vi "ReadIOValues gas.vi"(3 "error in":errorcluster, 5 "Output - Cluster gas":T1 {"GM TS-2[°C]" format="%.2g"; "GM TS-1 [°C]" format="%.4g"; "GM DS-1 [bar]" format="%.4g"; "GM DS-2 [bar]" format="%.2g"; "GM GZ-1 [imp]" format="%.2g"}) -> (0 "error out":errorcluster, 2 "Output - Cluster gas":T1 {"GM TS-2[°C]" format="%.2g"; "GM TS-1 [°C]" format="%.4g"; "GM DS-1 [bar]" format="%.4g"; "GM DS-2 [bar]" format="%.2g"; "GM GZ-1 [imp]" format="%.2g"})   [LabVIEW 2011]
uses:
  Output - Cluster gas.ctl
  gas_values.ctl
  <vilib>/functionblocks/Counter/Count Up/Count Up.vi
  <vilib>/functionblocks/FB Core/FB Core.xnode
  <vilib>/functionblocks/NI_FunctionBlock Libraries.lvlib
panel:
  # "qualitätsmessung"
  # "quantitätsmessung"
  # "qualitätsmessung"
  # "quantitätsmessung"
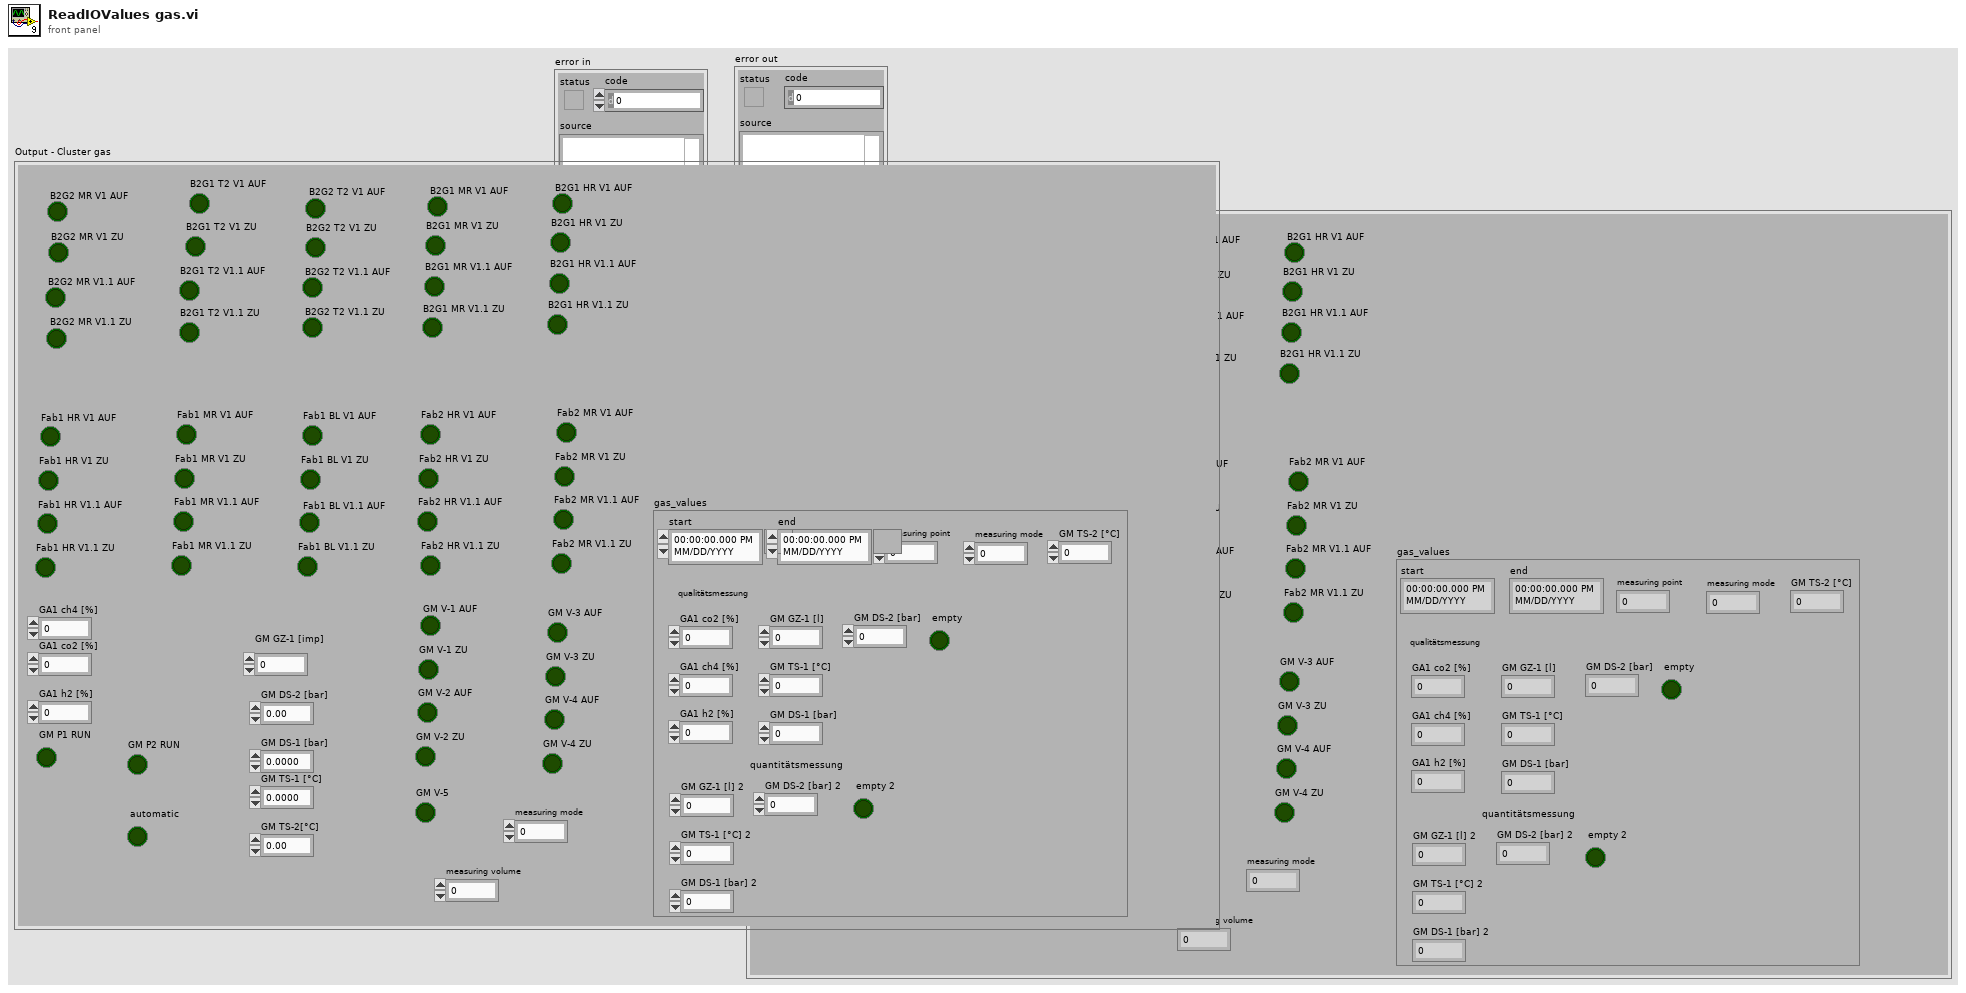
[diagram p1: front panel]
types:
  T1 = typedef "Output - Cluster gas.ctl" = cluster{"B2G2 MR V1.1 AUF":bool, "B2G2 MR V1.1 ZU":bool, "B2G2 MR V1 AUF":bool, "B2G2 MR V1 ZU":bool, "B2G1 T2 V1 AUF":bool, "B2G1 T2 V1 ZU":bool, "B2G1 T2 V1.1 AUF":bool, "B2G1 T2 V1.1 ZU":bool, "B2G2 T2 V1 AUF":bool, "B2G2 T2 V1 ZU":bool, "B2G2 T2 V1.1 ZU":bool, "B2G2 T2 V1.1 AUF":bool, "B2G1 MR V1 AUF":bool, "B2G1 MR V1 ZU":bool, "B2G1 MR V1.1 AUF":bool, "B2G1 MR V1.1 ZU":bool, "B2G1 HR V1 AUF":bool, "B2G1 HR V1 ZU":bool, "B2G1 HR V1.1 AUF":bool, "B2G1 HR V1.1 ZU":bool, "Fab1 HR V1 AUF":bool, "Fab1 HR V1 ZU":bool, "Fab1 HR V1.1 AUF":bool, "Fab1 HR V1.1 ZU":bool, "Fab1 MR V1 AUF":bool, "Fab1 MR V1 ZU":bool, "Fab1 MR V1.1 AUF":bool, "Fab1 MR V1.1 ZU":bool, "Fab1 BL V1 AUF":bool, "Fab1 BL V1 ZU":bool, "Fab1 BL V1.1 AUF":bool, "Fab1 BL V1.1 ZU":bool, "Fab2 HR V1 AUF":bool, "Fab2 HR V1 ZU":bool, "Fab2 HR V1.1 AUF":bool, "Fab2 HR V1.1 ZU":bool, "Fab2 MR V1 AUF":bool, "Fab2 MR V1 ZU":bool, "Fab2 MR V1.1 AUF":bool, "Fab2 MR V1.1 ZU":bool, "GA1 ch4 [%]":dbl, "GA1 co2 [%]":dbl, "GA1 h2 [%]":dbl, "GM P1 RUN":bool, "GM V-1 AUF":bool, "GM V-1 ZU":bool, "GM V-2 AUF":bool, "GM V-2 ZU":bool, "GM V-3 AUF":bool, "GM V-3 ZU":bool, "GM V-4 AUF":bool, "GM V-4 ZU":bool, "GM P2 RUN":bool, "GM GZ-1 [imp]":u32, "GM DS-2 [bar]":dbl, "GM DS-1 [bar]":dbl, "GM TS-1 [°C]":dbl, "GM TS-2[°C]":dbl, "gas_values":T2, "measuring mode":u8, "GM V-5":bool, "measuring volume":dbl, "automatic":bool}
  T2 = typedef "gas_values.ctl" = cluster{"start":timestamp, "GM DS-2 [bar]":dbl, "GA1 ch4 [%]":dbl, "GA1 co2 [%]":dbl, "GA1 h2 [%]":dbl, "GM DS-1 [bar]":dbl, "GM TS-1 [°C]":dbl, "GM TS-2 [°C]":dbl, "GM GZ-1 [l]":dbl, "measuring point":u8, "end":timestamp, "empty":bool, "GM GZ-1 [l] 2":dbl, "GM TS-1 [°C] 2":dbl, "GM DS-1 [bar] 2":dbl, "GM DS-2 [bar] 2":dbl, "empty 2":bool, "measuring mode":u8}
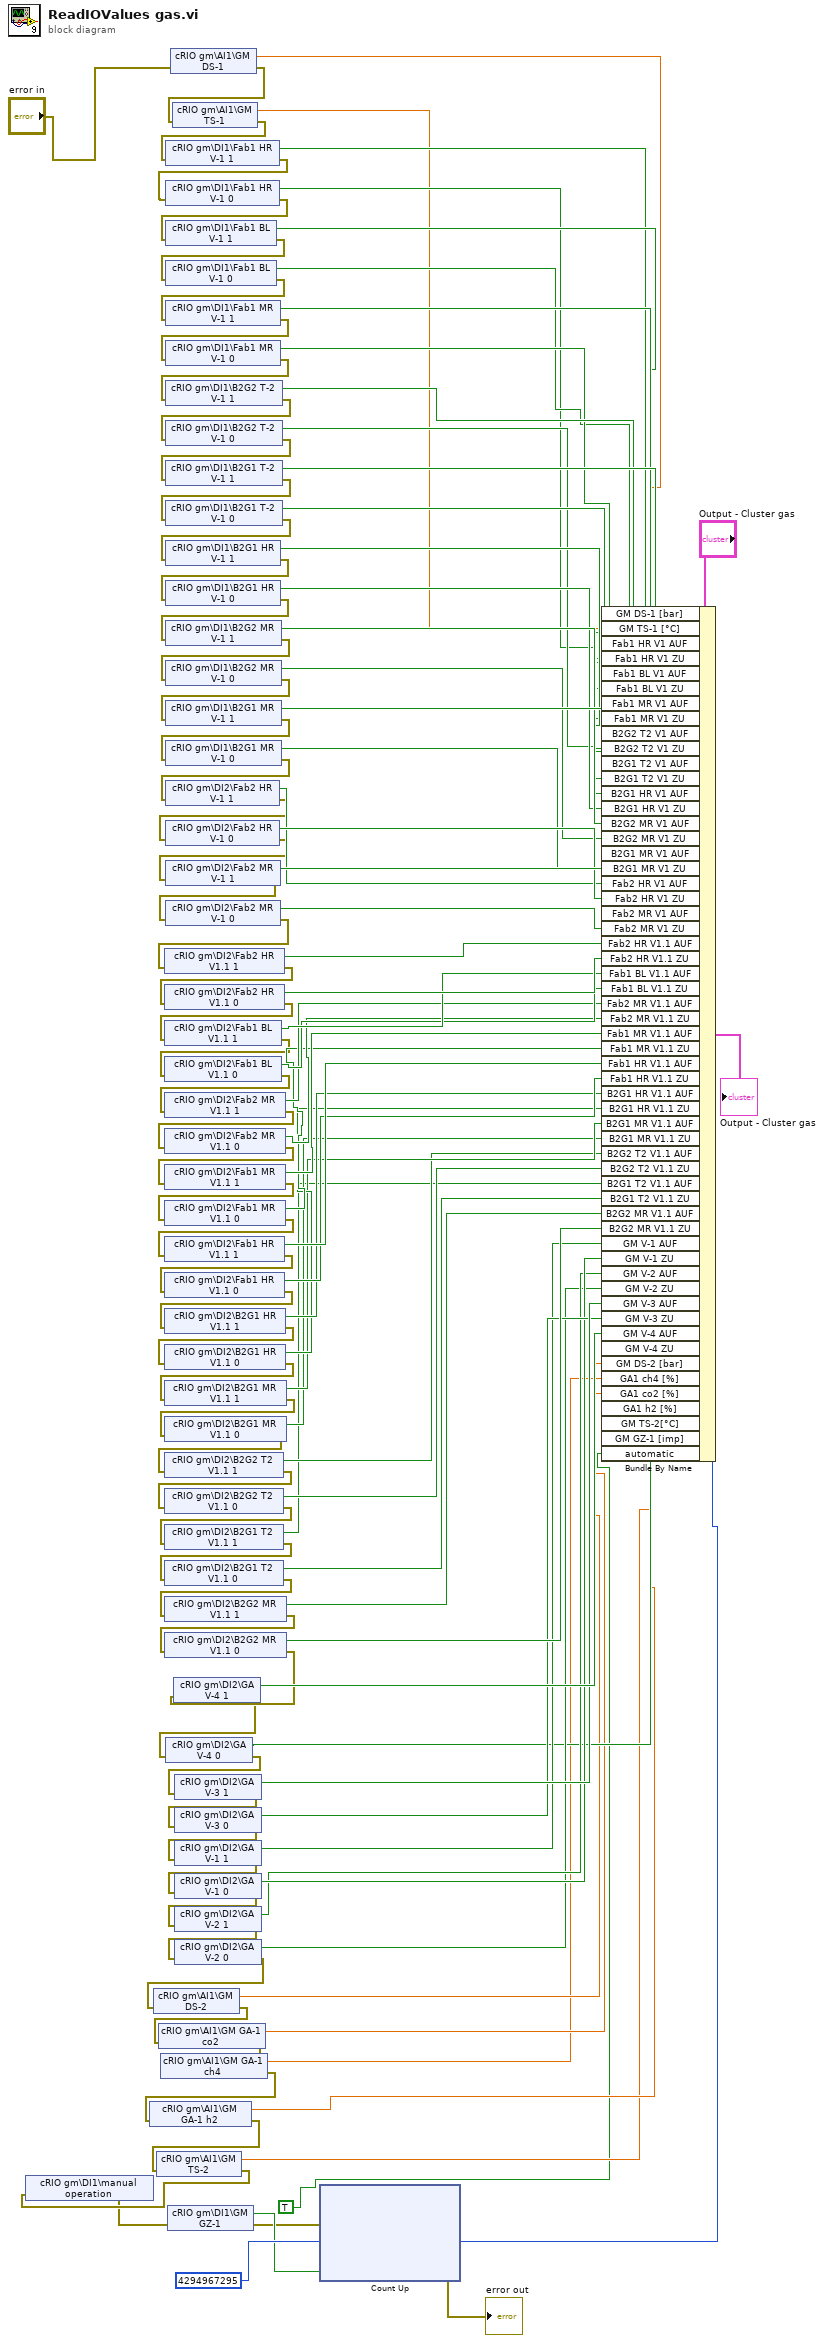
[diagram p0: block diagram]
diagram:
  n1 = shared-variable "cRIO gm\\AI1\\GM DS-1"(error in="error in") -> (w5:dbl, error out=w7:errorcluster)
  n2 = shared-variable "cRIO gm\\AI1\\GM TS-1"(error in=w7) -> (w4:dbl, error out=w6:errorcluster)
  n3 = shared-variable "cRIO gm\\DI1\\Fab1 HR V-1 1"(error in=w6) -> (w9:bool, error out=w44:errorcluster)
  n4 = shared-variable "cRIO gm\\DI1\\Fab1 HR V-1 0"(error in=w44) -> (w10:bool, error out=w43:errorcluster)
  n5 = shared-variable "cRIO gm\\DI1\\Fab1 BL V-1 1"(error in=w43) -> (w11:bool, error out=w42:errorcluster)
  n6 = shared-variable "cRIO gm\\DI1\\Fab1 BL V-1 0"(error in=w42) -> (w12:bool, error out=w41:errorcluster)
  n7 = shared-variable "cRIO gm\\DI1\\Fab1 MR V-1 1"(error in=w41) -> (w13:bool, error out=w40:errorcluster)
  n8 = shared-variable "cRIO gm\\DI1\\Fab1 MR V-1 0"(error in=w40) -> (w14:bool, error out=w39:errorcluster)
  n9 = shared-variable "cRIO gm\\DI1\\B2G2 T-2 V-1 1"(error in=w39) -> (w15:bool, error out=w38:errorcluster)
  n10 = shared-variable "cRIO gm\\DI1\\B2G2 T-2 V-1 0"(error in=w38) -> (w16:bool, error out=w37:errorcluster)
  n11 = shared-variable "cRIO gm\\DI1\\B2G1 T-2 V-1 1"(error in=w37) -> (w17:bool, error out=w36:errorcluster)
  n12 = shared-variable "cRIO gm\\DI1\\B2G1 T-2 V-1 0"(error in=w36) -> (w18:bool, error out=w35:errorcluster)
  n13 = shared-variable "cRIO gm\\DI1\\B2G1 HR V-1 1"(error in=w35) -> (w19:bool, error out=w34:errorcluster)
  n14 = shared-variable "cRIO gm\\DI1\\B2G1 HR V-1 0"(error in=w34) -> (w20:bool, error out=w33:errorcluster)
  n15 = shared-variable "cRIO gm\\DI1\\B2G2 MR V-1 1"(error in=w33) -> (w21:bool, error out=w32:errorcluster)
  n16 = shared-variable "cRIO gm\\DI1\\B2G2 MR V-1 0"(error in=w32) -> (w22:bool, error out=w31:errorcluster)
  n17 = shared-variable "cRIO gm\\DI1\\B2G1 MR V-1 1"(error in=w31) -> (w24:bool, error out=w30:errorcluster)
  n18 = shared-variable "cRIO gm\\DI1\\B2G1 MR V-1 0"(error in=w30) -> (w23:bool, error out=w29:errorcluster)
  n19 = shared-variable "cRIO gm\\DI2\\Fab2 HR V-1 1"(error in=w29) -> (w45:bool, error out=w28:errorcluster)
  n20 = shared-variable "cRIO gm\\DI2\\Fab2 HR V-1 0"(error in=w28) -> (w46:bool, error out=w27:errorcluster)
  n21 = shared-variable "cRIO gm\\DI2\\Fab2 MR V-1 1"(error in=w27) -> (w47:bool, error out=w26:errorcluster)
  n22 = shared-variable "cRIO gm\\DI2\\Fab2 MR V-1 0"(error in=w26) -> (w48:bool, error out=w25:errorcluster)
  n23 = shared-variable "cRIO gm\\DI2\\Fab2 HR V1.1 1"(error in=w25) -> (w118:bool, error out=w98:errorcluster)
  n24 = shared-variable "cRIO gm\\DI2\\Fab2 HR V1.1 0"(error in=w98) -> (w117:bool, error out=w97:errorcluster)
  n25 = shared-variable "cRIO gm\\DI2\\Fab1 BL V1.1 1"(error in=w97) -> (w116:bool, error out=w96:errorcluster)
  n26 = shared-variable "cRIO gm\\DI2\\Fab1 BL V1.1 0"(error in=w96) -> (w115:bool, error out=w95:errorcluster)
  n27 = shared-variable "cRIO gm\\DI2\\Fab2 MR V1.1 1"(error in=w95) -> (w114:bool, error out=w94:errorcluster)
  n28 = shared-variable "cRIO gm\\DI2\\Fab2 MR V1.1 0"(error in=w94) -> (w113:bool, error out=w93:errorcluster)
  n29 = shared-variable "cRIO gm\\DI2\\Fab1 MR V1.1 1"(error in=w93) -> (w112:bool, error out=w92:errorcluster)
  n30 = shared-variable "cRIO gm\\DI2\\Fab1 MR V1.1 0"(error in=w92) -> (w111:bool, error out=w91:errorcluster)
  n31 = shared-variable "cRIO gm\\DI2\\Fab1 HR V1.1 1"(error in=w91) -> (w110:bool, error out=w90:errorcluster)
  n32 = shared-variable "cRIO gm\\DI2\\Fab1 HR V1.1 0"(error in=w90) -> (w109:bool, error out=w89:errorcluster)
  n33 = shared-variable "cRIO gm\\DI2\\B2G1 HR V1.1 1"(error in=w89) -> (w108:bool, error out=w88:errorcluster)
  n34 = shared-variable "cRIO gm\\DI2\\B2G1 HR V1.1 0"(error in=w88) -> (w107:bool, error out=w87:errorcluster)
  n35 = shared-variable "cRIO gm\\DI2\\B2G1 MR V1.1 1"(error in=w87) -> (w106:bool, error out=w86:errorcluster)
  n36 = shared-variable "cRIO gm\\DI2\\B2G1 MR V1.1 0"(error in=w86) -> (w105:bool, error out=w85:errorcluster)
  n37 = shared-variable "cRIO gm\\DI2\\B2G2 T2 V1.1 1"(error in=w85) -> (w104:bool, error out=w84:errorcluster)
  n38 = shared-variable "cRIO gm\\DI2\\B2G2 T2 V1.1 0"(error in=w84) -> (w103:bool, error out=w83:errorcluster)
  n39 = shared-variable "cRIO gm\\DI2\\B2G1 T2 V1.1 1"(error in=w83) -> (w102:bool, error out=w82:errorcluster)
  n40 = shared-variable "cRIO gm\\DI2\\B2G1 T2 V1.1 0"(error in=w82) -> (w101:bool, error out=w81:errorcluster)
  n41 = shared-variable "cRIO gm\\DI2\\B2G2 MR V1.1 1"(error in=w81) -> (w100:bool, error out=w80:errorcluster)
  n42 = shared-variable "cRIO gm\\DI2\\B2G2 MR V1.1 0"(error in=w80) -> (w99:bool, error out=w72:errorcluster)
  n43 = shared-variable "cRIO gm\\DI2\\GA V-4 1"(error in=w72) -> (w79:bool, error out=w65:errorcluster)
  n44 = shared-variable "cRIO gm\\DI2\\GA V-4 0"(error in=w65) -> (w66:bool, error out=w64:errorcluster)
  n45 = shared-variable "cRIO gm\\DI2\\GA V-3 1"(error in=w64) -> (w78:bool, error out=w71:errorcluster)
  n46 = shared-variable "cRIO gm\\DI2\\GA V-3 0"(error in=w71) -> (w77:bool, error out=w70:errorcluster)
  n47 = shared-variable "cRIO gm\\DI2\\GA V-1 1"(error in=w70) -> (w76:bool, error out=w69:errorcluster)
  n48 = shared-variable "cRIO gm\\DI2\\GA V-1 0"(error in=w69) -> (w75:bool, error out=w68:errorcluster)
  n49 = shared-variable "cRIO gm\\DI2\\GA V-2 1"(error in=w68) -> (w74:bool, error out=w67:errorcluster)
  n50 = shared-variable "cRIO gm\\DI2\\GA V-2 0"(error in=w67) -> (w73:bool, error out=w63:errorcluster)
  n51 = shared-variable "cRIO gm\\AI1\\GM DS-2"(error in=w63) -> (w59:dbl, error out=w62:errorcluster)
  n52 = shared-variable "cRIO gm\\AI1\\GM GA-1 co2"(error in=w62) -> (w58:dbl, error out=w61:errorcluster)
  n53 = shared-variable "cRIO gm\\AI1\\GM GA-1 ch4"(error in=w61) -> (w57:dbl, error out=w60:errorcluster)
  n54 = shared-variable "cRIO gm\\AI1\\GM GA-1 h2"(error in=w60) -> (w56:dbl, error out=w54:errorcluster)
  n55 = shared-variable "cRIO gm\\AI1\\GM TS-2"(error in=w54) -> (w55:dbl, error out=w3:errorcluster)
  n56 = shared-variable "cRIO gm\\DI1\\manual operation"(error in=w3) -> (error out=w2:errorcluster)  [unwired: 1 out]
  n57 = shared-variable "cRIO gm\\DI1\\GM GZ-1"(error in=w2) -> (w52:bool, error out=w50:errorcluster)
  n58 = xnode "Count Up"("error in"=w50, "preset value"=u32 4294967295, "count up"=w52) -> ("error out"=→"error out":errorcluster, "counter value"=w51:u32)  [unwired: 1 in, 1 out]
  n59 = Bundle By Name(cluster="Output - Cluster gas", "GM DS-1 [bar]"=w5, "GM TS-1 [°C]"=w4, "Fab1 HR V1 AUF"=w9, "Fab1 HR V1 ZU"=w10, "Fab1 BL V1 AUF"=w11, "Fab1 BL V1 ZU"=w12, "Fab1 MR V1 AUF"=w13, "Fab1 MR V1 ZU"=w14, "B2G2 T2 V1 AUF"=w15, "B2G2 T2 V1 ZU"=w16, "B2G1 T2 V1 AUF"=w17, "B2G1 T2 V1 ZU"=w18, "B2G1 HR V1 AUF"=w19, "B2G1 HR V1 ZU"=w20, "B2G2 MR V1 AUF"=w21, "B2G2 MR V1 ZU"=w22, "B2G1 MR V1 AUF"=w24, "B2G1 MR V1 ZU"=w23, "Fab2 HR V1 AUF"=w45, "Fab2 HR V1 ZU"=w46, "Fab2 MR V1 AUF"=w47, "Fab2 MR V1 ZU"=w48, "Fab2 HR V1.1 AUF"=w118, "Fab2 HR V1.1 ZU"=w117, "Fab1 BL V1.1 AUF"=w116, "Fab1 BL V1.1 ZU"=w115, "Fab2 MR V1.1 AUF"=w114, "Fab2 MR V1.1 ZU"=w113, "Fab1 MR V1.1 AUF"=w112, "Fab1 MR V1.1 ZU"=w111, "Fab1 HR V1.1 AUF"=w110, "Fab1 HR V1.1 ZU"=w109, "B2G1 HR V1.1 AUF"=w108, "B2G1 HR V1.1 ZU"=w107, "B2G1 MR V1.1 AUF"=w106, "B2G1 MR V1.1 ZU"=w105, "B2G2 T2 V1.1 AUF"=w104, "B2G2 T2 V1.1 ZU"=w103, "B2G1 T2 V1.1 AUF"=w102, "B2G1 T2 V1.1 ZU"=w101, "B2G2 MR V1.1 AUF"=w100, "B2G2 MR V1.1 ZU"=w99, "GM V-1 AUF"=w76, "GM V-1 ZU"=w75, "GM V-2 AUF"=w74, "GM V-2 ZU"=w73, "GM V-3 AUF"=w78, "GM V-3 ZU"=w77, "GM V-4 AUF"=w79, "GM V-4 ZU"=w66, "GM DS-2 [bar]"=w59, "GA1 ch4 [%]"=w57, "GA1 co2 [%]"=w58, "GA1 h2 [%]"=w56, "GM TS-2[°C]"=w55, "GM GZ-1 [imp]"=w51, "automatic"=TRUE ("manual operation")) -> (→"Output - Cluster gas":T1)
